vi "Get Autorange Bereiche Ausnahmen.vi"(11 "result string (Eingang)":string) -> (3 "result string (Ausgang)":string)   [LabVIEW 2020, in "Linearisierung v2.lvlib"]
uses:
  Linearisierung v2.lvlib
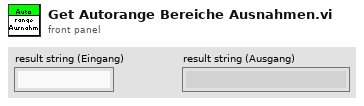
[diagram p1: front panel]
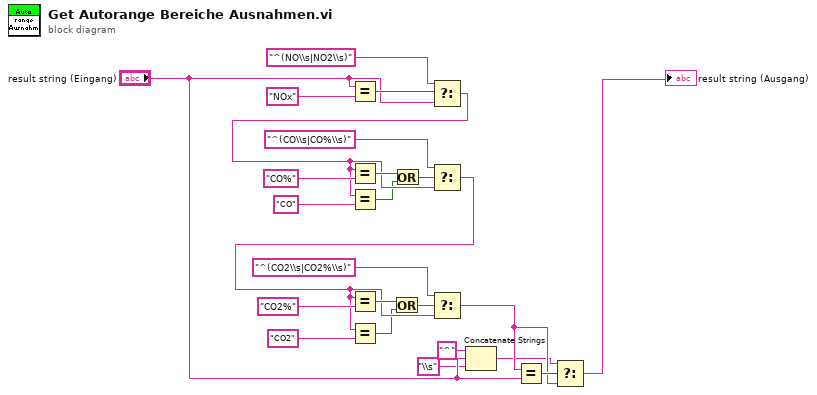
[diagram p0: block diagram]
diagram:
  n1 = Equal?(x="result string (Eingang)", y="NOx") -> (x = y?=w23:bool)
  n2 = Select(t="^(NO\\s|NO2\\s)", s=w23, f="result string (Eingang)") -> (s? t:f=w14:string)
  n3 = Equal?(x=w14, y="CO%") -> (x = y?=w15:bool)
  n4 = Equal?(x=w14, y="CO") -> (x = y?=w10:bool)
  n5 = Or(x=w15, y=w10) -> (x .or. y?=w11:bool)
  n6 = Select(t="^(CO\\s|CO%\\s)", s=w11, f=w14) -> (s? t:f=w12:string)
  n7 = Equal?(x=w12, y="CO2%") -> (x = y?=w18:bool)
  n8 = Equal?(x=w12, y="CO2") -> (x = y?=w8:bool)
  n9 = Or(x=w18, y=w8) -> (x .or. y?=w9:bool)
  n10 = Select(t="^(CO2\\s|CO2%\\s)", s=w9, f=w12) -> (s? t:f=w6:string)
  n11 = Concatenate Strings("^" ("String"), "result string (Eingang)", "\\s" ("String")) -> (w3:string)
  n12 = Equal?(x=w6, y="result string (Eingang)") -> (x = y?=w7:bool)
  n13 = Select(t=w3, s=w7, f=w6) -> (s? t:f=→"result string (Ausgang)":string)
